vi "LCAIO Get Output Sw Scaling Param.vi"(8 "error in (no error)":errorcluster caption="Fehler (Eingang, kein Fehler)", 11 "Output Channel Handle":i64) -> (0 "error out":errorcluster caption="Fehler (Ausgang)", 2 "Scaling Offset":dbl, 3 "Scaling Factor":dbl)   [LabVIEW 2021, in "labbCAN_AnalogIO_API.lvlib"]
doc: "LCAIO_Func long LCAIO_CALL LCAIO_GetOutputSwScalingParam(dev_hdl OutChanHdl,\n double *pScalingFactor,\n double *pScalingOffset);"
uses:
  labbCAN_AnalogIO_API.lvlib
  labbCAN_AnalogIO_API.dll
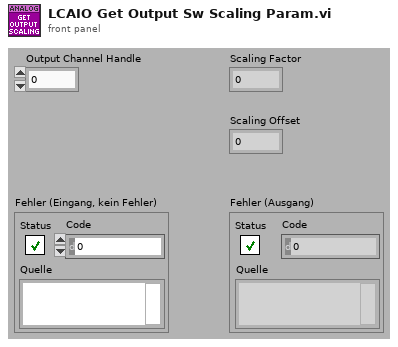
[diagram p1: front panel]
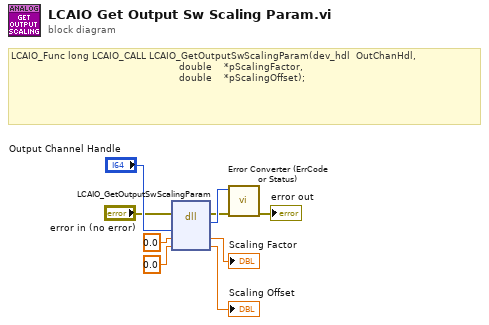
[diagram p0: block diagram]
diagram:
  # "LCAIO_Func long LCAIO_CALL LCAIO_GetOutputSwScalingParam(dev_hdl  OutChanHdl,\n                                                        double    *pScalingFactor,\n                                                        double    *pScalingOffset);"
  n1 = dll-call lib="C:/Users/olaja/AppData/Local/CETONI_SDK/labbCAN_AnalogIO_API.*" fn="LCAIO_GetOutputSwScalingParam"(error in="error in (no error)", "Output Channel Handle"="Output Channel Handle", "Scaling Factor"=0.0, "Scaling Offset"=0.0) -> (error out=w2:errorcluster, "Rückgabetyp"=w3:i32, "Scaling Factor"=→"Scaling Factor":dbl, "Scaling Offset"=→"Scaling Offset":dbl)  [unwired: 3 in, 1 out]
  n2 = call "Error Converter (ErrCode or Status).vi"("error in (no error)"=w2, "error code"=w3) -> ("error out"=→"error out":errorcluster)  [unwired: 9 in]
